vi "CIE2T-Compute Max SPL.vi"(0 "Acoustic System":string, 1 "f1 (kHz)":dbl, 2 "f2 (kHz)":dbl, 5 "Probe mic gain (dB)":dbl, 7 "Attenuation (dB)":dbl[](array[numeric]), 9 "df (kHz)":dbl, 11 "error in (no error)":errorcluster, 12 "+Freq. Mag of FFT":dbl[](array[numeric]) min=0.0 max=127.0 format="%.2f") -> (4 "Max SPL1":dbl, 6 "Max SPL2":dbl, 15 "error out":errorcluster)   [LabVIEW 2020]
uses:
  Utility VIs/Math VIs/dB to Linear (scalar).vi
  SubVIs/Calibration Globals.vi
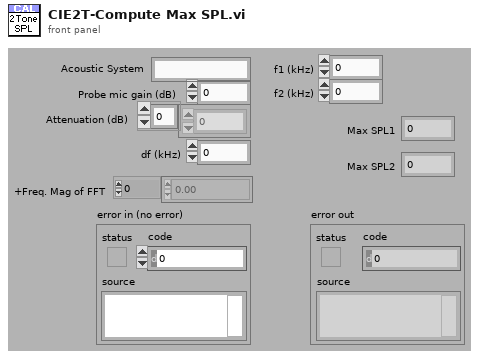
[diagram p1: front panel]
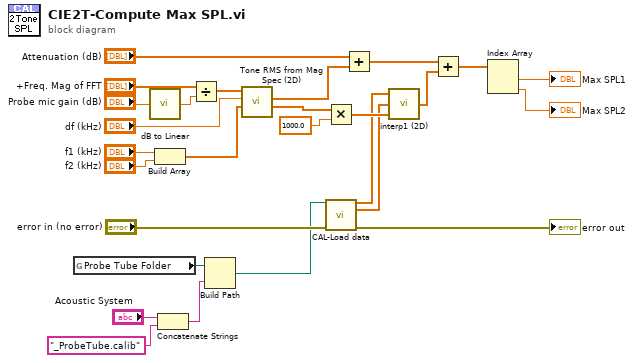
[diagram p0: block diagram]
diagram:
  n1 = global read "Calibration Globals.vi" "Probe Tube Folder"() -> (w6:path)
  n2 = call-poly "dB to Linear.vi"("dB"="Probe mic gain (dB)") -> ("linear"=w19:dbl)
  n3 = Build Array("f1 (kHz)", "f2 (kHz)") -> (w22:dbl[])
  n4 = Concatenate Strings("Acoustic System", "_ProbeTube.calib" ("string")) -> (w7:string)
  n5 = Divide(x="+Freq. Mag of FFT", y=w19) -> (x/y=w20:dbl[])
  n6 = Build Path(base path=w6, name or relative path=w7) -> (appended path=w4:path)
  n7 = call "Tone RMS from Mag Spec (2D).vi"("Frequency (kHz)"=w22, "df (kHz)"="df (kHz)", "Magnitude (dB)"=w20) -> ("Fpeak (kHz)"=w17:dbl[], "RMS (dB)"=w14:dbl[])  [unwired: 6 in, 1 out]
  n8 = Multiply(x=w17, y=1000.0) -> (x*y=w10:dbl[])
  n9 = call "CAL-Load data.vi"("user path"=w4, "error in (no error)"="error in (no error)") -> ("Frequency (Hz)"=w3:dbl[], "Mag"=w2:dbl[], "error out"=→"error out":errorcluster)  [unwired: 6 in, 5 out]
  n10 = Add(x="Attenuation (dB)", y=w14) -> (x+y=w15:dbl[])
  n11 = call "interp1 (2D).vi"("X"=w3, "Y"=w2, "U"=w10) -> ("V"=w16:dbl[])  [unwired: 2 in]
  n12 = Add(x=w15, y=w16) -> (x+y=w11:dbl[])
  n13 = Index Array(array=w11) -> (element #1=→"Max SPL1":dbl, element #2=→"Max SPL2":dbl)  [unwired: 2 in]
